vi "Run Tests.vi"(7 "Run Tests In Parallel? (T)":bool=TRUE, 8 "error in (no error)":errorcluster, 10 "Report Output path":path, 11 "Project, Library, or Test Class Path":path) -> (0 "error out":errorcluster, 1 "Aggregate Result":string, 2 "Output":string)   [LabVIEW 2020, in "Execution API.lvclass"]
doc: "Run all tests from the selected path programmatically. The path may point to a .lvclass, .lvlib, or .lvproj file. Results are generated at the provided Report Output Path. If the file extenssion is .txt, a plain text file is generated, and if it is .xml, an JUnit compatible .xml report is generated."
uses:
  Execution API.lvclass
  Core/Result/Status.ctl
  Core/Result/Type.ctl
  Core/Result/Result.lvlib
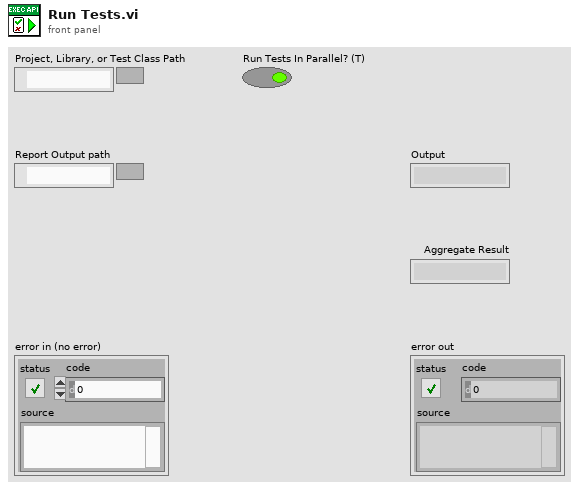
[diagram p1: front panel]
types:
  T1 = typedef "Result.lvlib/Status.ctl" = enum16{"", "Passed", "Failed", "Error", "Skipped", "Setup Error", "Broken", "Teardown Error"}
  T2 = typedef "Result.lvlib/Type.ctl" = enum16{"Test Case", "Test Suite", "Test Run", "Pass", "Fail", "Skip", "Pass if", "Fail if", "Pass if Error", "Fail if Error", "Pass if Equal", "Fail if Equal"}
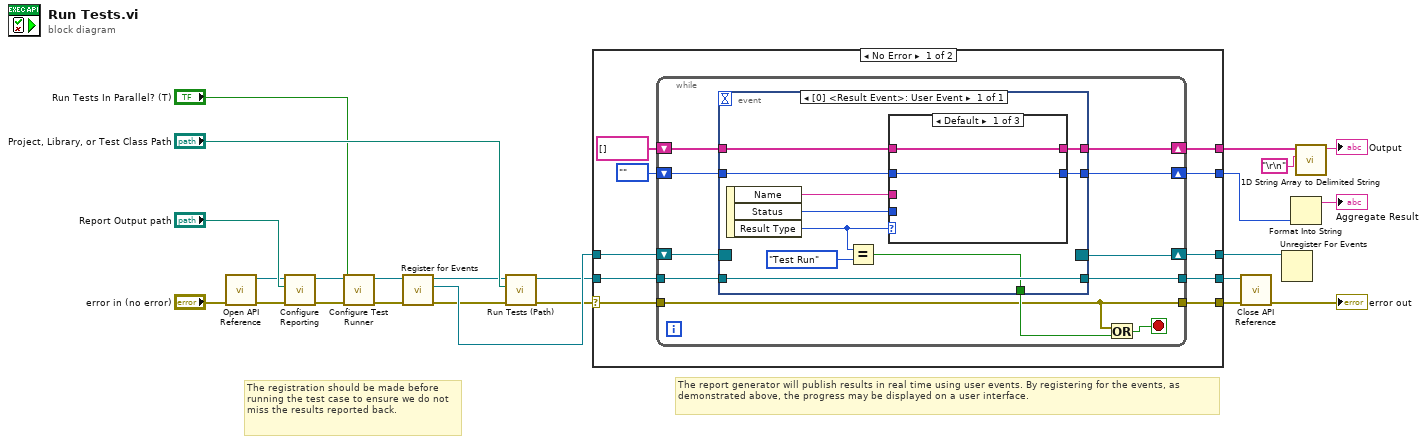
[diagram p0: block diagram]
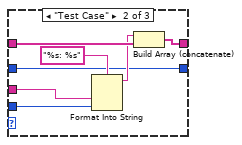
[diagram p2: hidden frame]
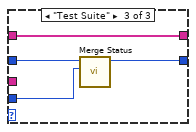
[diagram p3: hidden frame]
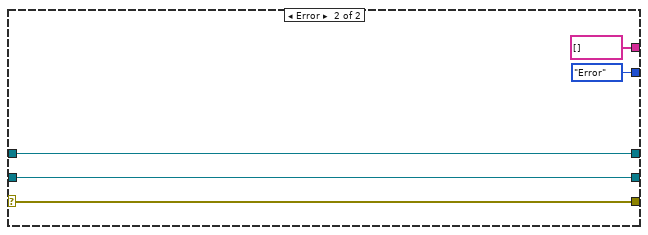
[diagram p4: hidden frame]
diagram:
  # "The registration should be made before running the test case to ensure we do not miss the results reported back."
  # "The report generator will publish results in real time using user events. By registering for the events, as demonstrated above, the progress may be displayed on a user interface."
  n1 = call "Open API Reference.vi"("error in (no error)"="error in (no error)") -> ("error out"=w12:errorcluster, "Execution API Out"=w16:refnum<class "Execution API.lvclass">)  [unwired: 9 in]
  n2 = call "Configure Reporting.vi"("error in (no error)"=w12, "Path"="Report Output path", "Execution API In"=w16) -> ("error out"=w14:errorcluster, "Execution API Out"=w13:refnum<class "Execution API.lvclass">)  [unwired: 7 in]
  n3 = call "Configure Test Runner.vi"("error in (no error)"=w14, "Run Tests In Parallel?"="Run Tests In Parallel? (T)", "Execution API In"=w13) -> ("error out"=w15:errorcluster, "Execution API Out"=w17:refnum<class "Execution API.lvclass">)  [unwired: 7 in]
  n4 = call "Register for Events.vi"("error in (no error)"=w15, "Execution API In"=w17) -> ("error out"=w9:errorcluster, "Event Registration"=w11:refnum<event-registration>, "Execution API Out"=w10:refnum<class "Execution API.lvclass">)  [unwired: 7 in]
  n5 = call "Run Tests (Path).vi"("error in (no error)"=w9, "Project or Class Path"="Project, Library, or Test Class Path", "Execution API In"=w10) -> ("error out"=w5:errorcluster, "Execution API Out"=w4:refnum<class "Execution API.lvclass">)  [unwired: 7 in]
  n6 = case shown="No Error" w5 {
    selector: w5 -> [w33 w73]
    tunnel: w11 -> [w34 w71]
    tunnel: w4 -> [w32 w72]
    tunnel: [w30 w73] -> w6
    tunnel: [w29 w72] -> w7
    tunnel: [w28 w71] -> w19
    tunnel: [w27 string[] []] -> w22
    tunnel: [w25 Status."Error" ("Status")] -> w2
    frame No Error {
      n7 = while {
        tunnel: w33 -> [w37]
        tunnel: w32 -> [w43]
        tunnel: [w41] -> w29
        tunnel: [w37] -> w30
        shift-right: [w38] -> w27
        shift-left: string[] [] -> [w45]
        shift-right: [w42] -> w28
        shift-left: w34 -> [w44]
        shift-right: [w35] -> w25
        shift-left: Status."" ("Status") -> [w36]
        stop <- w40 stop-if-true
        n8 = event shown="[0] <Result Event>: User Event" {
          selector: w44 -> [_]
          dyn-events: [_] -> w42
          timeout: _ -> [_]
          tunnel: w45 -> [w50]
          tunnel: w43 -> [w55]
          tunnel: [w55] -> w41
          tunnel: [w53] -> w39
          tunnel: [w49] -> w38
          tunnel: w36 -> [w47]
          tunnel: [w46] -> w35
          event User Event {
            n9 = event-data() -> ("Name"=w52:string, "Status"=w51:T1, "Result Type"=w48:T2)  [unwired: 1 in]
            n10 = Equal?(x=w48, y=Type."Test Run") -> (x = y?=w53:bool)
            n11 = case shown="Default" w48 {
              tunnel: w52 -> [_ w63 _]
              tunnel: w51 -> [_ w62 w66]
              tunnel: w50 -> [w57 w61 w68]
              tunnel: [w57 w59 w68] -> w49
              tunnel: w47 -> [w56 w58 w67]
              tunnel: [w56 w58 w65] -> w46
              frame Default {
              }
              frame "Test Case" {
                n12 = Format Into String(format string="%s: %s", w63, w62) -> (resulting string=w60:string)  [unwired: 2 in, 1 out]
                n13 = Build Array (concatenate)(w60, w61) -> (w59:string[])
              }
              frame "Test Suite" {
                n14 = call "Merge Status.vi"("New"=w66, "Current"=w67) -> ("Status"=w65:T1)  [unwired: 9 in]
              }
            }
          }
        }
        n15 = Or(x=w37, y=w39) -> (x .or. y?=w40:bool)
      }
    }
    frame Error {
    }
  }
  n16 = call "Close API Reference.vi"("error in (no error)"=w6, "Execution API In"=w7) -> ("error out"=→"error out":errorcluster)  [unwired: 9 in]
  n17 = Unregister For Events(event registration refnum=w19) -> ()  [unwired: 1 in, 1 out]
  n18 = Format Into String(w2) -> (resulting string=→"Aggregate Result":string)  [unwired: 3 in, 1 out]
  n19 = call <vilib>:"1D String Array to Delimited String.vi"("delimiter"="\r\n", "string array"=w22) -> ("delimited string"=→"Output":string)  [unwired: 9 in]
